vi "Test NI USB-6501.vi"   [LabVIEW 2020, in "NI USB-6501.lvclass"]
uses:
  NI USB-6501.lvclass
  Path Control/Measurements Specific Paths.ctl
  Path Control/PathControl.lvclass
types:
  T1 = typedef "PathControl.lvclass/Measurements Specific Paths.ctl" = enum16{"No calibration", "Harmonics", "IMD", "S Parameter", "AM-AM", "MCCW-ACLR", "DC", "LCR", "Power Meter GUI", "RF Power"}
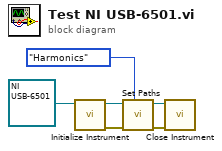
[diagram p0: block diagram]
diagram:
  n1 = call-dynamic "Initialize Instrument.vi"("NI USB-6501 in"=refnum<class "NI USB-6501.lvclass"> refnum) -> ("error out"=w2:errorcluster, "NI USB-6501 out"=w4:refnum<class "NI USB-6501.lvclass">)  [unwired: 9 in]
  n2 = call-dynamic "Set Paths.vi"("Measurement specific paths"=Measurements_Specific_Paths."Harmonics" ("Measurement specfic paths"), "error in (no error)"=w2, "NI USB-6501 in"=w4) -> ("error out"=w1:errorcluster, "NI USB-6501 out"=w3:refnum<class "NI USB-6501.lvclass">)  [unwired: 7 in]
  n3 = call-dynamic "Close Instrument.vi"("error in (no error)"=w1, "NI USB-6501 in"=w3) -> ()  [unwired: 8 in, 2 out]
